vi "toStringSpectrum.vi"(2 "value_in":u8[](array[numeric]), 3 "dim_y":i32, 4 "dim_x":i32) -> (0 "setpoint":string[](array[string]), 1 "value_out":string[](array[string]))   [LabVIEW 2014, in "tango.lvlib"]
uses:
  tango.lvlib
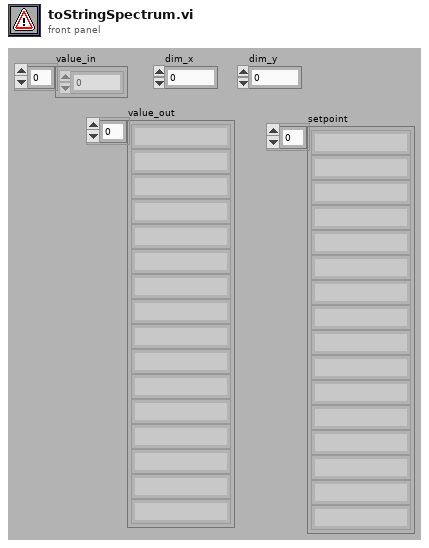
[diagram p1: front panel]
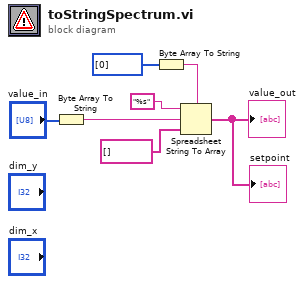
[diagram p0: block diagram]
diagram:
  n1 = Byte Array To String(unsigned byte array="value_in") -> (string=w2:string)
  n2 = Byte Array To String(unsigned byte array=u8[] [0]) -> (string=w4:string)
  n3 = Spreadsheet String To Array(delimiter (Tab)=w4, format string="%s", spreadsheet string=w2, array type (2D Dbl)=string[] []) -> (array=→"value_out" →"setpoint":string[])
